vi "Creators Is Created Event.vi"(10 "Created Event Alias":string, 11 "Base Event in":refnum<class "Base Event.lvclass">) -> (2 "Is Created Event?":bool, 3 "Base Event out":refnum<class "Base Event.lvclass">)   [LabVIEW 2021, in "jettl.lvlib" / "Base Event.lvlib" / "Base Event.lvclass"]
uses:
  Base Event.lvclass
  C:/git/jettl/src/jettl/jettl/jettl.lvclass
  Base Event.lvclass/Base Event.ctl
  Queue Mailbox/Queue Mailbox.lvlib
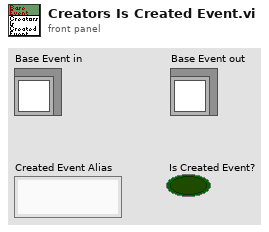
[diagram p1: front panel]
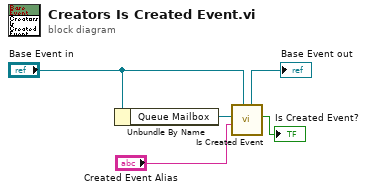
[diagram p0: block diagram]
diagram:
  n1 = Unbundle By Name("Base Event in") -> ("Queue Mailbox"=w3:refnum<data-value>)
  n2 = call "Is Created Event.vi"("jettl in"="Base Event in", "Created Event Alias"="Created Event Alias", "Queue Mailbox"=w3) -> ("Is Created Event?"=→"Is Created Event?":bool, "jettl out"=→"Base Event out":refnum<class "Base Event.lvclass">)  [unwired: 7 in]
